vi "DAQmx Create Channel (AI-Current-Basic).vi"(0 "task in":refnum<k21>, 1 "maximum value":dbl=0.01 format="%0.5f", 2 "minimum value":dbl=-0.01 format="%0.5f", 3 "input terminal configuration":i32(ring)=-1 items=["default"=-1, "RSE"=10083, "NRSE"=10078, "Differential"=10106, "Pseudodifferential"=12529], 5 "physical channels":tag, 7 "name to assign":string, 8 "external shunt resistor value":dbl=249.0 format="%0.2f", 9 "units":i32(ring)=10342 items=["Amps"=10342, "From Custom Scale"=10065], 11 "error in":errorcluster, 12 "custom scale name":tag, 14 "shunt resistor location":i32(ring)=-1 items=["default"=-1, "Internal"=10200, "External"=10167]) -> (4 "task out":refnum<k21>, 15 "error out":errorcluster)   [LabVIEW 2013]
doc: "Creates channel(s) to measure current."
uses:
  C:/Program Files/National Instruments/LabVIEW 2013/resource/objmgr/daqmx.rc
panel:
  # "input limits"
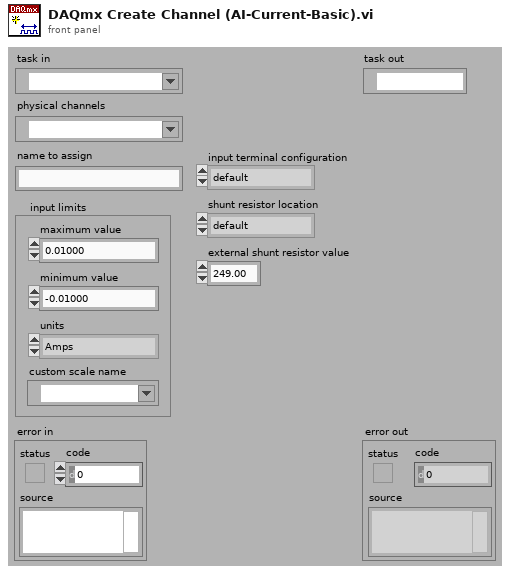
[diagram p1: front panel]
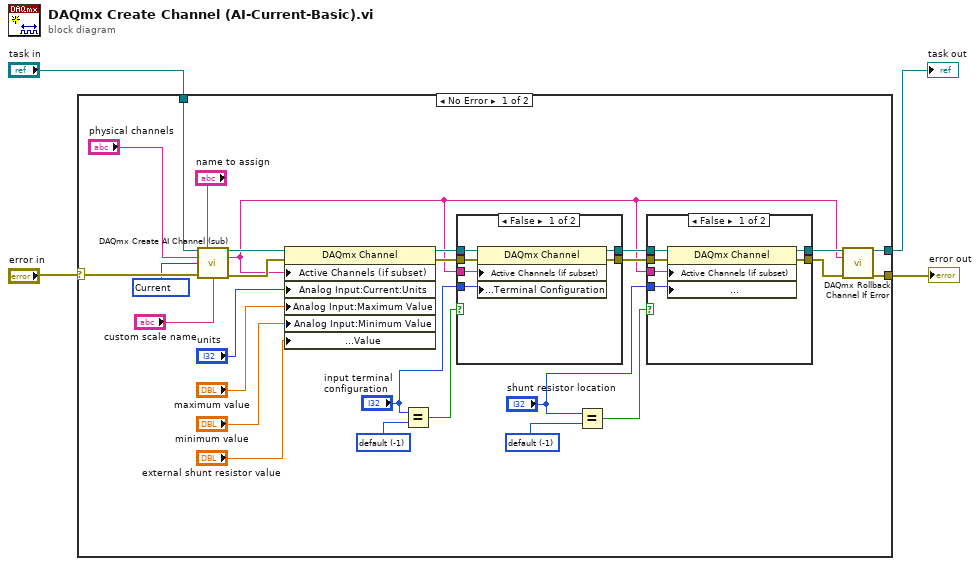
[diagram p0: block diagram]
diagram:
  n1 = case shown="No Error" "error in" {
    selector: "error in" -> [w30 w49]
    tunnel: [w13 w49] -> w4
    tunnel: [w14 w48] -> w3
    tunnel: "task in" -> [w29 w48]
    frame No Error {
      w7 = -1 items=["default"=-1, "Internal"=10200, "External"=10167] ("shunt resistor location")
      w17 = -1 items=["default"=-1, "differential"=10106, "RSE"=10083, "NRSE"=10078] ("input terminal configuration")
      w20 = 10134 items=["Voltage"=10322, "Current"=10134, "More:Voltage:Custom with Excitation"=10323, "More:Current:Custom with Excitation"=10136, "Frequency"=10181, "Period"=10257, "Resistance"=10278, "Temperature:Thermocouple"=10303, "Temperature:Thermistor"=10302, "Temperature:RTD"=10301, "Temperature:Built-in Sensor"=10311, "Strain Gage"=10300] ("measurement type")
      n2 = call "DAQmx Create AI Channel (sub).vi"("task in"=w29, "virtual channel name"="name to assign", "physical channel name"="physical channels", "measurement type"=w20, "error in"=w30, "custom scale"="custom scale name") -> ("task out"=w15:refnum<k21>, "channel names"=w8:string, "error out"=w28:errorcluster)  [unwired: 1 in, 6 out]
      n3 = property class="DAQmx Channel"(reference=w15, error in=w28, "Active Channels (if subset)"=w8, "Analog Input:Current:Units"="units", "Analog Input:Maximum Value"="maximum value", "Analog Input:Minimum Value"="minimum value", "Analog Input:General Properties:Signal Conditioning:Current Shunt Resistor:Value"="external shunt resistor value") -> (reference out=w23:refnum<k21>, error out=w22:errorcluster)
      n4 = Equal?(x="input terminal configuration", y=w17) -> (x = y?=w24:bool)
      n5 = case shown="False" w24 {
        tunnel: "input terminal configuration" -> [w42 _]
        tunnel: w23 -> [w40 w47]
        tunnel: [w45 w47] -> w12
        tunnel: w22 -> [w44 w46]
        tunnel: [w43 w46] -> w11
        tunnel: w8 -> [w41 _]
        frame False {
          n6 = property class="DAQmx Channel"(reference=w40, error in=w44, "Active Channels (if subset)"=w41, "Analog Input:General Properties:Input Configuration:Terminal Configuration"=w42) -> (reference out=w45:refnum<k21>, error out=w43:errorcluster)
        }
        frame True {
        }
      }
      n7 = Equal?(x="shunt resistor location", y=w7) -> (x = y?=w6:bool)
      n8 = case shown="False" w6 {
        tunnel: "shunt resistor location" -> [w34 _]
        tunnel: w12 -> [w32 w39]
        tunnel: [w37 w39] -> w10
        tunnel: w11 -> [w36 w38]
        tunnel: [w35 w38] -> w9
        tunnel: w8 -> [w33 _]
        frame False {
          n9 = property class="DAQmx Channel"(reference=w32, error in=w36, "Active Channels (if subset)"=w33, "Analog Input:General Properties:Signal Conditioning:Current Shunt Resistor:Location"=w34) -> (reference out=w37:refnum<k21>, error out=w35:errorcluster)
        }
        frame True {
        }
      }
      n10 = call "DAQmx Rollback Channel If Error.vi"("task in"=w10, "channel names"=w8, "error in"=w9) -> ("task out"=w14:refnum<k21>, "error out"=w13:errorcluster)  [unwired: 11 out]
    }
    frame Error {
    }
  }
  "error out" <- w4
  "task out" <- w3
